vi "terminate.vi"(8 "error in (no error)":errorcluster, 11 "GenericPlugin in":refnum<class "LightSourceMH110124MaiTai.lvclass">) -> (0 "error out":errorcluster, 3 "GenericPlugin out":refnum<class "LightSourceMH110124MaiTai.lvclass">)   [LabVIEW 2010, in "LightSourceMH110124MaiTai.lvclass"]
doc: "The dynamic dispatch version of this VI terminates the plug-in object by releasing all of its resources."
uses:
  LightSourceMH110124MaiTai.lvclass
  LightSourceScaffold/LightSourceScaffold/LightSourceScaffold.lvclass
  common/classes/ErrorController/ErrorController/class_data.vi
  common/classes/ErrorController/ErrorController/ErrorController.lvclass
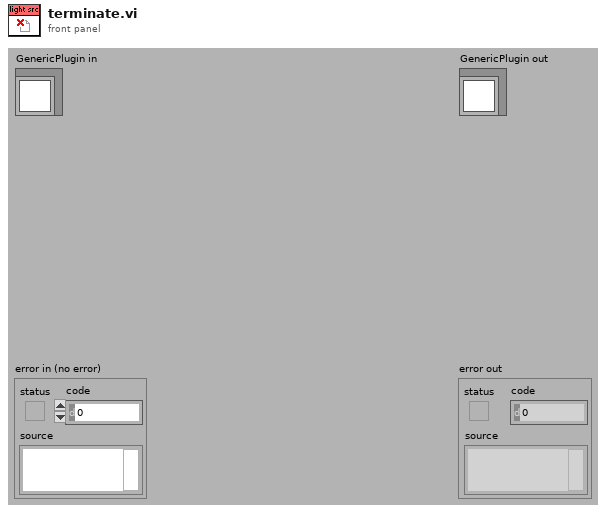
[diagram p1: front panel]
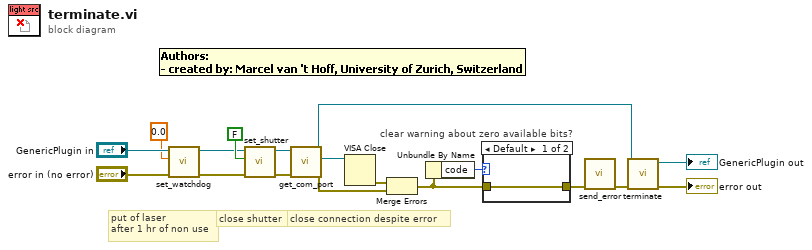
[diagram p0: block diagram]
diagram:
  # "put of laser\nafter 1 hr of non use"
  # "close shutter"
  # "close connection despite error"
  n1 = call-dynamic "set_watchdog.vi"("error in (no error)"="error in (no error)", "set timer"=dbl[unit] 0.0, "LightSourceMH110124MaiTai in"="GenericPlugin in") -> ("error out"=w2:errorcluster, "LightSourceMH110124MaiTai out"=w4:refnum<class "LightSourceMH110124MaiTai.lvclass">)  [unwired: 7 in]
  n2 = call-dynamic "set_shutter.vi"("error in (no error)"=w2, "shutter open?"=FALSE, "LightSourceMH110124MaiTai in"=w4) -> ("error out"=w10:errorcluster, "LightSourceMH110124MaiTai out"=w12:refnum<class "LightSourceMH110124MaiTai.lvclass">)  [unwired: 6 in, 1 out]
  n3 = call-dynamic "get_com_port.vi"("error in (no error)"=w10, "LightSourceMH110124MaiTai in"=w12) -> ("error out"=w9:errorcluster, "comm port"=w8:refnum<visa-resource-name>, "LightSourceMH110124MaiTai out"=w11:refnum<class "LightSourceMH110124MaiTai.lvclass">)  [unwired: 7 in]
  n4 = VISA Close(VISA resource name=w8) -> (error out=w14:errorcluster)  [unwired: 1 in]
  n5 = Merge Errors(w14, w9) -> (w16:errorcluster)
  n6 = Unbundle By Name(w16) -> ("code"=w15:i32)
  n7 = case "clear warning about zero available bits?" shown="Default" w15 {
    tunnel: [w19 _] -> w6
    tunnel: w16 -> [w19 _]
    frame Default {
    }
    frame 1073676294 {
    }
  }
  n8 = call "send_error.vi"("error in (no error)"=w6) -> ("error out"=w7:errorcluster)  [unwired: 10 in]
  n9 = call-parent "terminate.vi"("error in (no error)"=w7, "GenericPlugin in"=w11) -> ("error out"=→"error out":errorcluster, "GenericPlugin out"=→"GenericPlugin out":refnum<class "LightSourceMH110124MaiTai.lvclass">)  [unwired: 8 in]
